vi "Extract Single Pixel Velocity(SubVI).vi"(6 "Velocity Component 2":T1, 8 "limit":sgl, 9 "Rectangle":cluster{dbl, dbl, dbl, dbl, dbl}, 11 "Velocity Component 1":T1) -> (2 "Vector sum Comp 2":dbl, 3 "Vector sum Comp 1":dbl)   [LabVIEW 2014]
uses:
  <vilib>/vision/Image Controls.llb/IMAQ Image.ctl
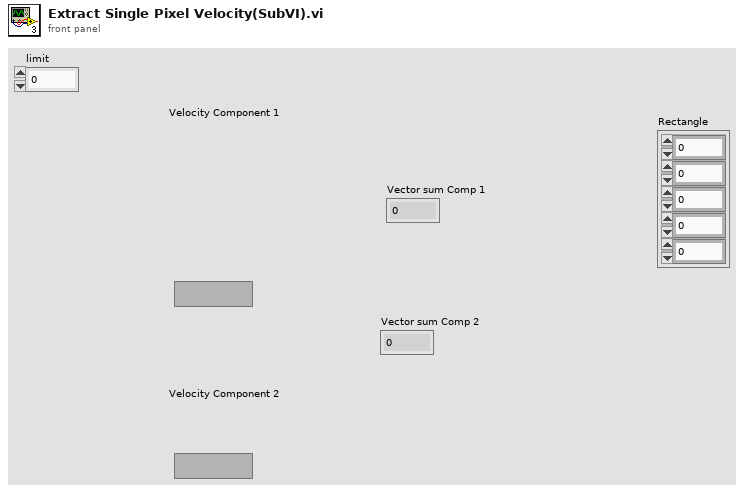
[diagram p1: front panel]
types:
  T1 = typedef "IMAQ Image.ctl" = refnum<image>
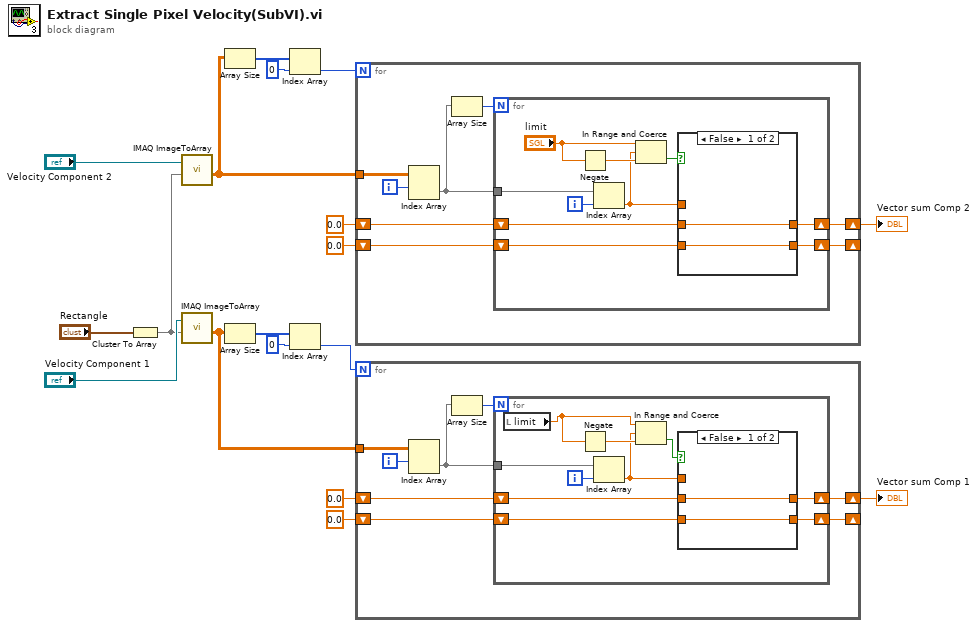
[diagram p0: block diagram]
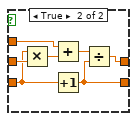
[diagram p2: hidden frame]
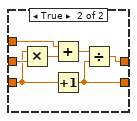
[diagram p3: hidden frame]
diagram:
  n1 = Cluster To Array(cluster="Rectangle") -> (array=w15:dbl[])
  n2 = call "IMAQ ImageToArray"("Optional Rectangle"=w15, "Image"="Velocity Component 2") -> ("Image Pixels (Float)"=w9:sgl[][])  [unwired: 2 in, 4 out]
  n3 = call "IMAQ ImageToArray"("Optional Rectangle"=w15, "Image"="Velocity Component 1") -> ("Image Pixels (Float)"=w2:sgl[][])  [unwired: 2 in, 4 out]
  n4 = Array Size(array=w9) -> (size(s)=w12:i32[])
  n5 = Array Size(array=w2) -> (size(s)=w14:i32[])
  n6 = Index Array(array=w12, index=0) -> (element=w8:i32)
  n7 = Index Array(array=w14, index=0) -> (element=w3:i32)
  n8 = for {
    N: w8 -> [_]
    tunnel: w9 -> [w26]
    shift-right: [w21] -> w7
    shift-left: 0.0 -> [w23]
    shift-right: [w19] -> _
    shift-left: 0.0 -> [w20]
    i -> [w25]
    n9 = Index Array(array=w26, index (row)=w25) -> (element=w24:sgl[])  [unwired: 1 in]
    n10 = Array Size(array=w24) -> (size(s)=w22:i32)
    n11 = for {
      N: w22 -> [_]
      tunnel: w24 -> [w36]
      shift-right: [w29] -> w21
      shift-left: w23 -> [w30]
      shift-right: [w27] -> w19
      shift-left: w20 -> [w28]
      i -> [w35]
      n12 = Negate(x="limit") -> (-x=w34:sgl)
      n13 = Index Array(array=w36, index=w35) -> (element=w31:sgl)
      n14 = In Range and Coerce(upper limit="limit", x=w31, lower limit=w34) -> (In Range?=w32:bool)  [unwired: 1 out]
      n15 = case shown="False" w32 {
        tunnel: w31 -> [_ w43]
        tunnel: w30 -> [w37 w45]
        tunnel: [w37 w41] -> w29
        tunnel: w28 -> [w38 w40]
        tunnel: [w38 w39] -> w27
        frame False {
        }
        frame True {
          n16 = Multiply(x=w40, y=w45) -> (x*y=w44:dbl)
          n17 = Add(x=w43, y=w44) -> (x+y=w42:dbl)
          n18 = Increment(x=w40) -> (x+1=w39:dbl)
          n19 = Divide(x=w42, y=w39) -> (x/y=w41:dbl)
        }
      }
    }
  }
  "Vector sum Comp 2" <- w7
  n20 = for {
    N: w3 -> [_]
    tunnel: w2 -> [w53]
    shift-right: [w48] -> w1
    shift-left: 0.0 -> [w50]
    shift-right: [w46] -> _
    shift-left: 0.0 -> [w47]
    i -> [w52]
    n21 = Index Array(array=w53, index (row)=w52) -> (element=w51:sgl[])  [unwired: 1 in]
    n22 = Array Size(array=w51) -> (size(s)=w49:i32)
    n23 = for {
      N: w49 -> [_]
      tunnel: w51 -> [w63]
      shift-right: [w57] -> w48
      shift-left: w50 -> [w58]
      shift-right: [w55] -> w46
      shift-left: w47 -> [w56]
      i -> [w62]
      n24 = local read "limit"() -> (w54:sgl)
      n25 = Negate(x=w54) -> (-x=w61:sgl)
      n26 = Index Array(array=w63, index=w62) -> (element=w59:sgl)
      n27 = In Range and Coerce(upper limit=w54, x=w59, lower limit=w61) -> (In Range?=w60:bool)  [unwired: 1 out]
      n28 = case shown="False" w60 {
        tunnel: w59 -> [_ w70]
        tunnel: w58 -> [w64 w72]
        tunnel: [w64 w68] -> w57
        tunnel: w56 -> [w65 w67]
        tunnel: [w65 w66] -> w55
        frame False {
        }
        frame True {
          n29 = Multiply(x=w67, y=w72) -> (x*y=w71:dbl)
          n30 = Add(x=w70, y=w71) -> (x+y=w69:dbl)
          n31 = Increment(x=w67) -> (x+1=w66:dbl)
          n32 = Divide(x=w69, y=w66) -> (x/y=w68:dbl)
        }
      }
    }
  }
  "Vector sum Comp 1" <- w1
